vi "Increment_Decrement by one Day.vi"(6 "Inc/Dec (No Change)":T1, 10 "Start Day":timestamp format="%<%x %.3X>T") -> (2 "End Day":timestamp format="%<%x %.3X>T")   [LabVIEW 2020, in "Time Management.lvlib"]
doc: "Returns the current day as a Timestamp. The timestamp will be rounded to the nearest factor of a day in seconds (86400). Since the beginning time in LabVIEW is January 1, 1904 12:00 am universal time, the specific time referenced will be related to your timezone referenced to univerasl time.\n\n08/2025, Erich Schlieper"
uses:
  Time Management.lvlib
  ENUM-Inc_Dec.ctl
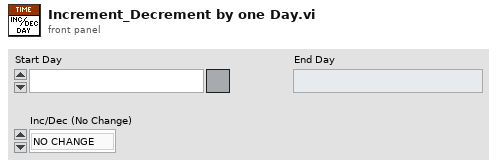
[diagram p1: front panel]
types:
  T1 = typedef "ENUM-Inc_Dec.ctl" = enum16{"NO CHANGE", "Increment", "Decrement"}
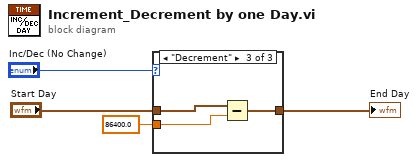
[diagram p0: block diagram]
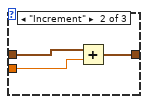
[diagram p3: hidden frame]
diagram:
  n1 = case shown="\"Decrement\"" "Inc/Dec (No Change)" {
    tunnel: [w5 w7 w10] -> w3
    tunnel: "Start Day" -> [w5 w8 w11]
    tunnel: 86400.0 ("x") -> [_ w6 w9]
    frame "NO CHANGE" {
    }
    frame "Increment" {
      n2 = Add(x=w8, y=w6) -> (x+y=w7:timestamp)
    }
    frame "Decrement" {
      n3 = Subtract(x=w11, y=w9) -> (x-y=w10:timestamp)
    }
  }
  "End Day" <- w3
